vi "Configure Scope.vi"(8 "error in (no error)":errorcluster, 10 "Trigger Level Source":i32, 11 "Scope in":refnum<k15>) -> (0 "error out":errorcluster, 3 "Scope out":refnum<k15> caption="Instrument Handle Out")   [LabVIEW 2023, in "Bode Plot - PXI.lvlib"]
doc: "Initializes and configures the Scope channels and the acquisition"
uses:
  Bode Plot - PXI.lvlib
  <instrlib>/niScope/Controls/niScope trigger source.ctl
  <instrlib>/niScope/Controls/niScope trigger coupling.ctl
  <instrlib>/niScope/Controls/niScope trigger slope.ctl
  <instrlib>/niScope/Controls/niScope vertical coupling.ctl
  <instrlib>/niScope/Configure/Trigger/niScope Configure Trigger Edge.vi
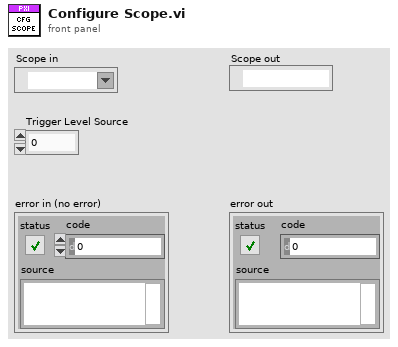
[diagram p1: front panel]
types:
  T1 = typedef "niScope trigger source.ctl" = string
  T2 = typedef "niScope trigger slope.ctl" = i32
  T3 = typedef "niScope trigger coupling.ctl" = u16
  T4 = typedef "niScope vertical coupling.ctl" = i32
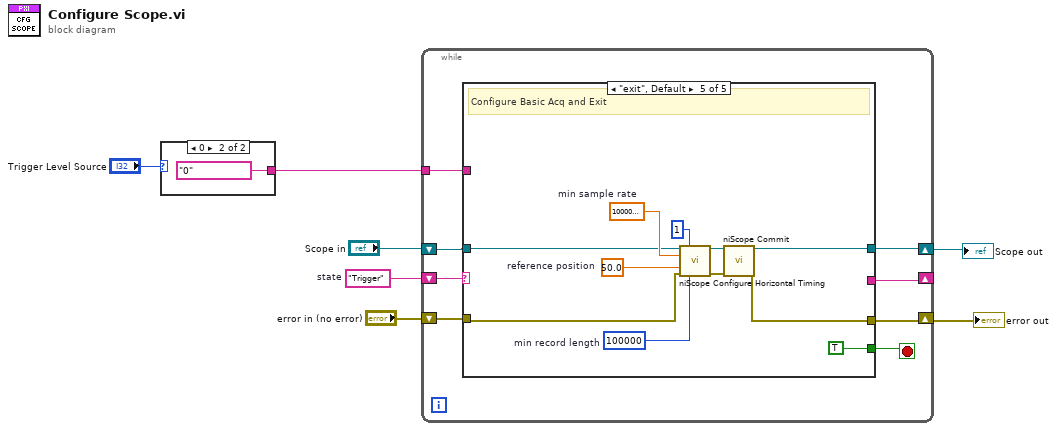
[diagram p0: block diagram]
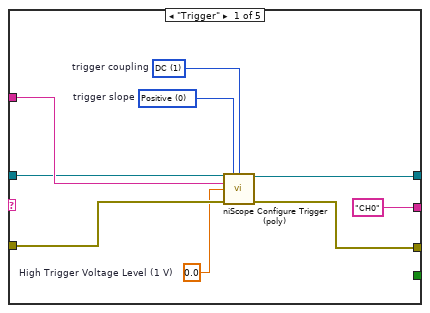
[diagram p2: hidden frame]
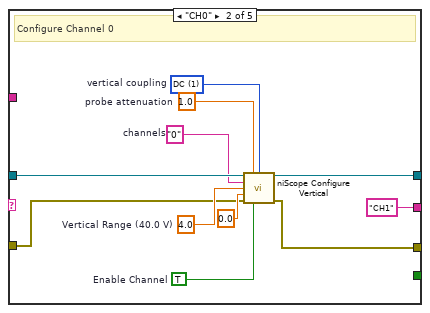
[diagram p3: hidden frame]
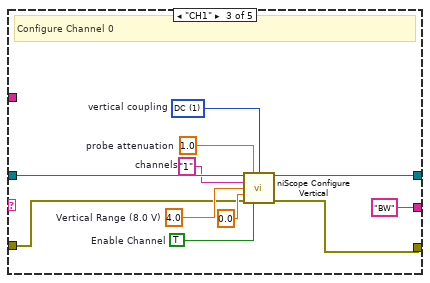
[diagram p4: hidden frame]
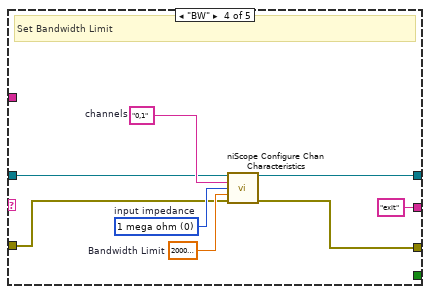
[diagram p5: hidden frame]
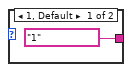
[diagram p6: hidden frame]
diagram:
  w6 = "Trigger"  # state
  n1 = case shown="0" "Trigger Level Source" {
    tunnel: [T1 "1" ("trigger source") T1 "0" ("trigger source")] -> w4
    frame 1, Default {
    }
    frame 0 {
    }
  }
  n2 = while {
    shift-right: [w13] -> _
    shift-left: w6 -> [w17]
    tunnel: w4 -> [w15]
    shift-right: [w12] -> w1
    shift-left: "Scope in" -> [w11]
    shift-right: [w14] -> w3
    shift-left: "error in (no error)" -> [w16]
    stop <- w10 stop-if-true
    n3 = case shown="\"exit\", Default" w17 {
      tunnel: w16 -> [w26 w30 w41 w52 w60]
      tunnel: w15 -> [w25 _ _ _ _]
      tunnel: w11 -> [w24 w36 w47 w55 w58]
      tunnel: [w20 w29 w40 w51 w65] -> w14
      tunnel: ["CH0" "CH1" "BW" "exit" _] -> w13
      tunnel: [w18 w27 w38 w49 w66] -> w12
      tunnel: [_ _ _ _ TRUE] -> w10
      frame "Trigger" {
        w21 = 0.0  # High Trigger Voltage Level (1 V)
        w22 = T2 0 items=["Positive", "Negative"]  # trigger slope
        w23 = T3 1 items=["AC"=0, "DC"=1, "HF Reject"=3, "LF Reject"=4, "AC Plus HF Reject"=1001]  # trigger coupling
        n4 = call-poly <instrlib>:"niScope Configure Trigger (poly).vi"("instrument handle"=w24, "trigger slope"=w22, "trigger coupling"=w23, "trigger source"=w25, "trigger level"=w21, "error in"=w26) -> ("instrument handle out"=w18:refnum<k15>, "error out"=w20:errorcluster)  [unwired: 8 in]
      }
      frame "CH0" {
        w34 = "0"  # channels
        w37 = T4 1 items=["AC", "DC", "Ground"]  # vertical coupling
        w35 = 1.0  # probe attenuation
        w33 = TRUE  # Enable Channel
        w32 = 4.0  # Vertical Range (40.0 V)
        # "Configure Channel 0"
        n5 = call <instrlib>:"niScope Configure Vertical.vi"("instrument handle"=w36, "probe attenuation"=w35, "vertical coupling"=w37, "channels"=w34, "vertical range"=w32, "vertical offset"=0.0, "error in"=w30, "channel enabled"=w33) -> ("instrument handle out"=w27:refnum<k15>, "error out"=w29:errorcluster)  [unwired: 6 in]
      }
      frame "CH1" {
        w45 = "1"  # channels
        w48 = T4 1 items=["AC", "DC", "Ground"]  # vertical coupling
        w46 = 1.0  # probe attenuation
        w44 = TRUE  # Enable Channel
        w43 = 4.0  # Vertical Range (8.0 V)
        # "Configure Channel 0"
        n6 = call <instrlib>:"niScope Configure Vertical.vi"("instrument handle"=w47, "probe attenuation"=w46, "vertical coupling"=w48, "channels"=w45, "vertical range"=w43, "vertical offset"=0.0, "error in"=w41, "channel enabled"=w44) -> ("instrument handle out"=w38:refnum<k15>, "error out"=w40:errorcluster)  [unwired: 6 in]
      }
      frame "BW" {
        w56 = "0,1"  # channels
        w54 = u32 0 items=["1 mega ohm"=0, "50 ohms"=2]  # input impedance
        w53 = 20000000.0  # Bandwidth Limit
        # "Set Bandwidth Limit"
        n7 = call <instrlib>:"niScope Configure Chan Characteristics.vi"("instrument handle"=w55, "channels"=w56, "input impedance"=w54, "maximum input frequency"=w53, "error in"=w52) -> ("instrument handle out"=w49:refnum<k15>, "error out"=w51:errorcluster)  [unwired: 9 in]
      }
      frame "exit", Default {
        w61 = 100000  # min record length
        w62 = 100000000.0  # min sample rate
        w63 = 50.0  # reference position
        # "Configure Basic Acq and Exit"
        n8 = call <instrlib>:"niScope Configure Horizontal Timing.vi"("instrument handle"=w58, "number of records"=1, "min sample rate"=w62, "reference position"=w63, "error in"=w60, "min record length"=w61) -> ("instrument handle out"=w59:refnum<k15>, "error out"=w57:errorcluster)  [unwired: 8 in]
        n9 = call <instrlib>:"niScope Commit.vi"("instrument handle"=w59, "error in"=w57) -> ("instrument handle out"=w66:refnum<k15>, "error out"=w65:errorcluster)  [unwired: 12 in]
      }
    }
  }
  "error out" <- w3
  "Scope out" <- w1
